vi "basic_serial_write_and_read_event.vi"() -> ()   [LabVIEW 2011]
uses:
  <vilib>/Instr/_visa.llb/VISA Configure Serial Port (Instr).vi
panel:
  out "Nbytes prev clear":u32
  out "Bytes read in response":u32
  out "Bytes written to Serial":u32
  out "iteration":i32
  in  "stop":bool
  in  "Write to Serial port now":bool
  in  "read":bool=TRUE
  in  "string to write":string="*IDN?"
  in  "write":bool=TRUE
  out "bytes read":u32=5
  out "read string":string
  in  "flow control":u16(ring) items=["None"=0, "XON/XOFF"=1, "RTS/CTS"=2, "DTR/DSR"=4]
  in  "stop bits":u16(ring)=10 items=["1.0"=10, "1.5"=15, "2.0"=20]
  in  "parity":u16(ring) items=["None", "Odd", "Even", "Mark", "Space"]
  in  "data bits":u16=8 min=5 max=8 step=1
  in  "VISA resource name":refnum<visa-resource-name>="COM1"
  in  "baud rate":u32=9600
  # "This program demonstrates a serial loop back with Teensyduino.\nEnter characters to write to serial port, click Go!\nThe response from the Teensy appears in 'read string'\n\nnote: you must first load firmware onto Teensy to execute serial loopback routine."
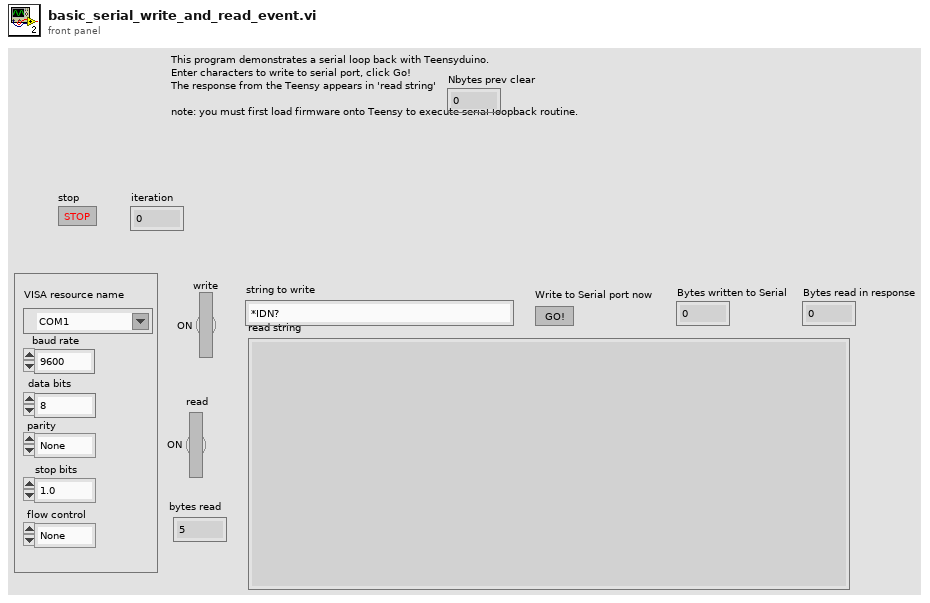
[diagram p1: front panel]
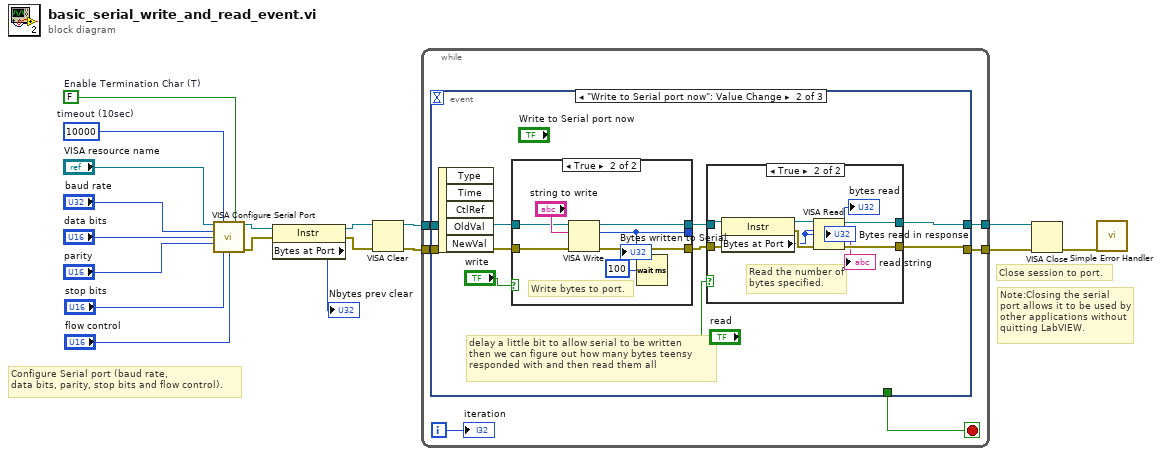
[diagram p0: block diagram]
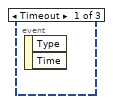
[diagram p2: hidden frame]
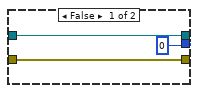
[diagram p3: hidden frame]
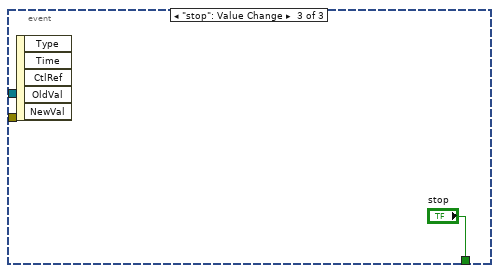
[diagram p5: hidden frame]
diagram:
  w11 = FALSE  # Enable Termination Char (T)
  w12 = u32 10000  # timeout (10sec)
  # "Note:Closing the serial port allows it to be used by other applications without\nquitting LabVIEW."
  # "Configure Serial port (baud rate,\ndata bits, parity, stop bits and flow control)."
  # "Close session to port."
  n1 = call-poly "VISA Configure Serial Port"("VISA resource name"="VISA resource name", "timeout (10sec)"=w12, "Enable Termination\nChar (T)"=w11, "baud rate (9600)"="baud rate", "data bits (8)"="data bits", "parity (0:none)"="parity", "stop bits (10: 1 bit)"="stop bits", "flow control (0:none)"="flow control") -> ("VISA resource name out"=w5:refnum<visa-resource-name>, "error out"=w4:errorcluster)  [unwired: 6 in]
  n2 = property class="Instr"(reference=w5, error in=w4) -> (reference out=w3:refnum<visa-resource-name>, error out=w2:errorcluster, "Bytes at Port"=→"Nbytes prev clear":u32)
  n3 = VISA Clear(VISA resource name=w3, error in (no error)=w2) -> (VISA resource name out=w6:refnum<visa-resource-name>, error out=w7:errorcluster)
  n4 = while {
    tunnel: w7 -> [w24]
    tunnel: w6 -> [w23]
    tunnel: [w22] -> w16
    tunnel: [w21] -> w15
    i -> [w19]
    stop <- w20 stop-if-true
    n5 = event shown="[1] \"Write to Serial port now\": Value Change" {
      selector: _ -> [_ _ _]
      dyn-events: _ -> [_ _ _]
      timeout: _ -> [_ _ _]
      tunnel: w24 -> [_ w29 _]
      tunnel: w23 -> [_ w28 _]
      tunnel: [_ w26 _] -> w22
      tunnel: [_ w27 _] -> w21
      tunnel: [_ _ "stop"] -> w20
      event Timeout {
        n6 = event-data() -> ()  [unwired: 1 in, 2 out]
      }
      event "Write to Serial port now": Value Change {
        # "delay a little bit to allow serial to be written\nthen we can figure out how many bytes teensy\nresponded with and then read them all"
        n7 = event-data() -> ()  [unwired: 1 in, 5 out]
        n8 = case shown="True" "write" {
          tunnel: [w35 w38] -> w31
          tunnel: w28 -> [w34 w41]
          tunnel: w29 -> [w35 w40]
          tunnel: [w34 w39] -> w25
          tunnel: [u32 0 ("Bytes at Port") w37] -> _
          frame False {
          }
          frame True {
            # "Write bytes to port."
            n9 = VISA Write(VISA resource name=w41, write buffer="string to write", error in (no error)=w40) -> (VISA resource name out=w39:refnum<visa-resource-name>, return count=w37:u32, error out=w38:errorcluster)
            "Bytes written to Serial" <- w37
            n10 = Wait (ms)(milliseconds to wait=u32 100) -> ()  [unwired: 1 out]
          }
        }
        n11 = case shown="True" "read" {
          tunnel: w31 -> [w44 w49]
          tunnel: [w44 w53] -> w26
          tunnel: [w43 w52] -> w27
          tunnel: w25 -> [w43 w45]
          frame False {
          }
          frame True {
            # "Read the number of bytes specified."
            n12 = property class="Instr"(reference=w45, error in=w49) -> (reference out=w46:refnum<visa-resource-name>, error out=w48:errorcluster, "Bytes at Port"=w47:u32)
            "Bytes read in response" <- w47
            n13 = VISA Read(VISA resource name=w46, byte count=w47, error in (no error)=w48) -> (VISA resource name out=w52:refnum<visa-resource-name>, read buffer=→"read string":string, return count=→"bytes read":u32, error out=w53:errorcluster)
          }
        }
      }
      event "stop": Value Change {
        n14 = event-data() -> ()  [unwired: 1 in, 5 out]
      }
    }
    "iteration" <- w19
  }
  n15 = VISA Close(VISA resource name=w15, error in (no error)=w16) -> (error out=w14:errorcluster)
  n16 = call <vilib>:"Simple Error Handler.vi"("error in (no error)"=w14) -> ()  [unwired: 4 in, 5 out]
